vi "Begin.vi"(8 "error in":errorcluster) -> (0 "error out":errorcluster)   [LabVIEW 2016]
doc: "Called before other user functions, this VI is expected to open initial I/O refnums, load in file data, and do all program initialization. Notice that the <B>error out</B> terminal is simply used for data flow. Wiring it to other structures or subVIs ensures that this VI runs first."
uses:
  <vilib>/Rock Robotics/SystemInterfaces/spilib/spi_bus.ctl
  <vilib>/Rock Robotics/WPI/SPI/WPI_SPIMode.ctl
  <vilib>/Rock Robotics/SystemInterfaces/DIO/FPGA_DIOPWMChannel.ctl
  <vilib>/Rock Robotics/WPI/SafetyOutput/WPI_SafetyOutputConfigMenu.ctl
  <vilib>/Rock Robotics/WPI/DriverStation/WPI_DriverStationRobotMode2.ctl
  <vilib>/Rock Robotics/WPI/Joystick/WPI_JoystickDeviceEnum.ctl
  <vilib>/Rock Robotics/SystemInterfaces/DIO/FPGA_DIOChannel.ctl
  <vilib>/Rock Robotics/WPI/Encoder/WPI_EncoderType.ctl
  NI WPI/WPI_SerialPort_USB.ctl
  <vilib>/Rock Robotics/WPI/ThirdParty/CanMotor/TalonSRX/WPI_CANTalonSRX_APIControlMode.ctl
  <vilib>/Rock Robotics/WPI/Solenoid/WPI_SolenoidChannel.ctl
  <vilib>/Rock Robotics/SystemInterfaces/i2clib/i2c_bus.ctl
  <vilib>/Rock Robotics/WPI/Solenoid/WPI_SolenoidValue.ctl
  Robot Global Data.vi
  <vilib>/Rock Robotics/Network Tables/NT Write String Array.vi
  <vilib>/Rock Robotics/WPI/Counter/WPI_CounterDigitalInputToDigitalSource.vi
  navX Library v2/IO/Open/Z900_navX_Open_Serial.vi
  <vilib>/Rock Robotics/WPI/Solenoid/WPI_SolenoidOpenSingle.vi
  <vilib>/Rock Robotics/WPI/MotorControl/WPI_MotorControlOpen VictorSP.vi
  <vilib>/Rock Robotics/WPI/RobotDrive/WPI_RobotDriveOpen4MotorWithVictorSP.vi
  <vilib>/Rock Robotics/WPI/Solenoid/WPI_SolenoidSetEnum.vi
  navX Library v2/navX Library v2.lvlib
  NI WPI/NI WPI Serial USB.lvlib
panel:
  in  "Chip Select Active High (F)":bool
  in  "Mode (3)":T1=enum."Mode 3 (Clk Idle High,Sample on Trailing)"
  in  "Clock Rate (Hz)":dbl=500000.0
  in  "SPI Bus":T2=enum."SPI On-Board, CS1"
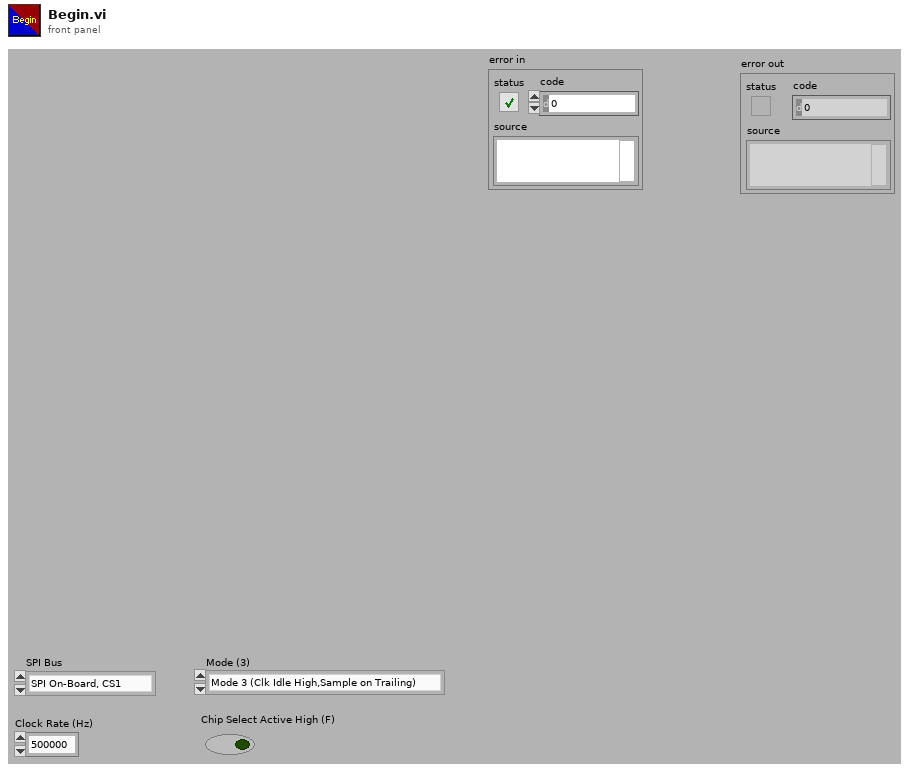
[diagram p1: front panel]
types:
  T1 = typedef "WPI_SPIMode.ctl" = enum16{"Mode 0 (Clk Idle Low,Sample on Leading)", "Mode 1 (Clk Idle Low,Sample on Trailing)", "Mode 2 (Clk Idle High,Sample on Leading)", "Mode 3 (Clk Idle High,Sample on Trailing)"}
  T2 = typedef "spi_bus.ctl" = enum16{"SPI On-Board, CS0", "SPI On-Board, CS1", "SPI On-Board, CS2", "SPI On-Board, CS3", "SPI MXP", "Invalid"}
  T3 = typedef "FPGA_DIOChannel.ctl" = enum8{"DIO 0", "DIO 1", "DIO 2", "DIO 3", "DIO 4", "DIO 5", "DIO 6", "DIO 7", "DIO 8", "DIO 9", "DIO MXP 0", "DIO MXP 1", "DIO MXP 2", "DIO MXP 3", "DIO MXP 4", "DIO MXP 5", "DIO MXP 6", "DIO MXP 7", "DIO MXP 8", "DIO MXP 9", "DIO MXP 10", "DIO MXP 11", "DIO MXP 12", "DIO MXP 13", "DIO MXP 14", "DIO MXP 15", "SPI Port CS1", "SPI Port CS2", "SPI Port CS3", "SPI Port MISO", "SPI Port MOSI", "Invalid"}
  T4 = typedef "WPI_SolenoidValue.ctl" = enum16{"Off", "On", "Forward", "Reverse"}
  T5 = typedef "i2c_bus.ctl" = enum16{"I2C On-Board", "I2C MXP", "Invalid"}
  T6 = typedef "WPI_SolenoidChannel.ctl" = enum8{"Solenoid 0", "Solenoid 1", "Solenoid 2", "Solenoid 3", "Solenoid 4", "Solenoid 5", "Solenoid 6", "Solenoid 7", "Invalid"}
  T7 = typedef "FPGA_DIOPWMChannel.ctl" = enum8{"PWM 0", "PWM 1", "PWM 2", "PWM 3", "PWM 4", "PWM 5", "PWM 6", "PWM 7", "PWM 8", "PWM 9", "PWM MXP 0", "PWM MXP 1", "PWM MXP 2", "PWM MXP 3", "PWM MXP 4", "PWM MXP 5", "PWM MXP 6", "PWM MXP 7", "PWM MXP 8", "PWM MXP 9", "Invalid"}
  T8 = typedef "WPI_JoystickDeviceEnum.ctl" = enum16{"USB 0", "USB 1", "USB 2", "USB 3", "USB 4", "USB 5"}
  T9 = typedef "WPI_CANTalonSRX_APIControlMode.ctl" = enum8{"Percent VBus", "Speed", "Position", "Slave", "Unchanged / Invalid", "Voltage Compensation", "Current", "Motion Profile", "Motion Magic"}
  T10 = typedef "NI WPI Serial USB.lvlib/WPI_SerialPort_USB.ctl" = enum16{"Onboard RS-232", "MXP TTL", "USB"}
  T11 = typedef "WPI_EncoderType.ctl" = enum16{"1x", "2x", "4x"}
  T12 = typedef "WPI_DriverStationRobotMode2.ctl" = enum16{"Autonomous Disabled", "Autonomous Enabled", "Teleop Disabled", "Teleop Enabled", "Disconnected", "Finish", "Test Disabled", "Test Enabled", "Emergency Stopped"}
  T13 = typedef "WPI_SafetyOutputConfigMenu.ctl" = enum16{"Enable", "Disable"}
  T14 = typedef "WPI_JoystickDevRef.ctl" = cluster{"Device":T8}
  T15 = typedef "WPI_I2CDevRef.ctl" = cluster{"DevStatus":errorcluster, "Device Address":u8, "Handle":i32, "I2C Bus":T5}
  T16 = typedef "WPI_MotorControlDeviceRef.ctl" = cluster{"DeviceStatus":errorcluster, "Type":T17, "PWM":cluster{"PWM Channel":T7, "DeadBand":T18}, "CAN":cluster{"Device Number":u8, "SetOutput VI Ref":variant, "GetOutput VI Ref":variant, "Enable VI Ref":variant, "Disable VI Ref":variant, "Data":variant}, "Invert":bool}
  T17 = typedef "WPI_MotorControlType.ctl" = enum16{"PWM", "CAN"}
  T18 = typedef "WPI_PWMDeadband.ctl" = cluster{"Name":string, "maxPositivePwm":i32, "minPositivePwm":i32, "centerPwm":i32, "maxNegativePwm":i32, "minNegativePwm":i32, "angularRange":u16}
  T19 = typedef "WPI_RobotDriveDevRef.ctl" = cluster{"DevStatus":errorcluster, "Motors[]":T16[], "Square Inputs":bool, "Max Output":dbl}
  T20 = typedef "WPI_SPIDevRef.ctl" = cluster{"DevStatus":errorcluster, "Handle":i32, "SPI Bus":T2}
  T21 = typedef "WPI_DigitalInputDevRef.ctl" = cluster{"DevStatus":errorcluster, "DIO Channel":T3}
  T22 = typedef "FPGA_CounterEncoderSourceConvertionLVSourceType.ctl" = cluster{"DevStatus":errorcluster, "AnalogTriggerMode?":bool, "DigitalMode":cluster{"DIO Channel":T23}, "AnalogTriggerMode":cluster{"AnalogTriggerIndex":T24, "OutputType":T25}}
  T23 = typedef "FPGA_DIODigitalSourceChannel.ctl" = enum8{"DIO 0", "DIO 1", "DIO 2", "DIO 3", "DIO 4", "DIO 5", "DIO 6", "DIO 7", "DIO 8", "DIO 9", "DIO MXP 0", "DIO MXP 1", "DIO MXP 2", "DIO MXP 3", "DIO MXP 4", "DIO MXP 5", "DIO MXP 6", "DIO MXP 7", "DIO MXP 8", "DIO MXP 9", "DIO MXP 10", "DIO MXP 11", "DIO MXP 12", "DIO MXP 13", "DIO MXP 14", "DIO MXP 15", "Disabled"}
  T24 = typedef "FPGA_AnalogTriggerIndex.ctl" = enum8{"Trig 0", "Trig 1", "Trig 2", "Trig 3", "Trig 4", "Trig 5", "Trig 6", "Trig 7", "Invalid"}
  T25 = typedef "FPGA_AnalogTriggerOutType.ctl" = enum16{"InWindow", "TriggerState", "Rising", "Falling"}
  T26 = typedef "WPI_EncoderDevRef.ctl" = cluster{"DevStatus":errorcluster, "EncoderIndex":T27, "CounterIndex":T28, "DistancePerCount":dbl, "Decoding Type":T11}
  T27 = typedef "FPGA_EncoderIdx.ctl" = enum8{"Enc 0", "Enc 1", "Enc 2", "Enc 3", "Enc 4", "Enc 5", "Enc 6", "Enc 7", "Invalid"}
  T28 = typedef "FPGA_CounterCtrSystemIndex.ctl" = enum8{"Ctr 0", "Ctr 1", "Ctr 2", "Ctr 3", "Ctr 4", "Ctr 5", "Ctr 6", "Ctr 7", "Invalid"}
  T29 = typedef "navX Library v2.lvlib/Z900_navX_DeviceTypeDef.ctl" = cluster{"Interface":cluster{"Protocol":T30, "Update Rate (4Hz-100Hz)":u8, "navX Open TypeDef":variant}, "Notify Packet":refnum<notifier>, "Loop VI Refnum":refnum<vi>, "Ready to Close Occurrence Refnum":refnum<k4>}
  T30 = typedef "navX Library v2.lvlib/Z900_navX_ProtocolTypeDef.ctl" = enum16{"SERIAL", "I2C", "SPI"}
  T31 = typedef "WPI_SolenoidDevRef.ctl" = cluster{"DevStatus":errorcluster, "Pneumatics Control Module":u8, "Forward Solenoid Channel":T6, "Reverse Solenoid Channel":T6}
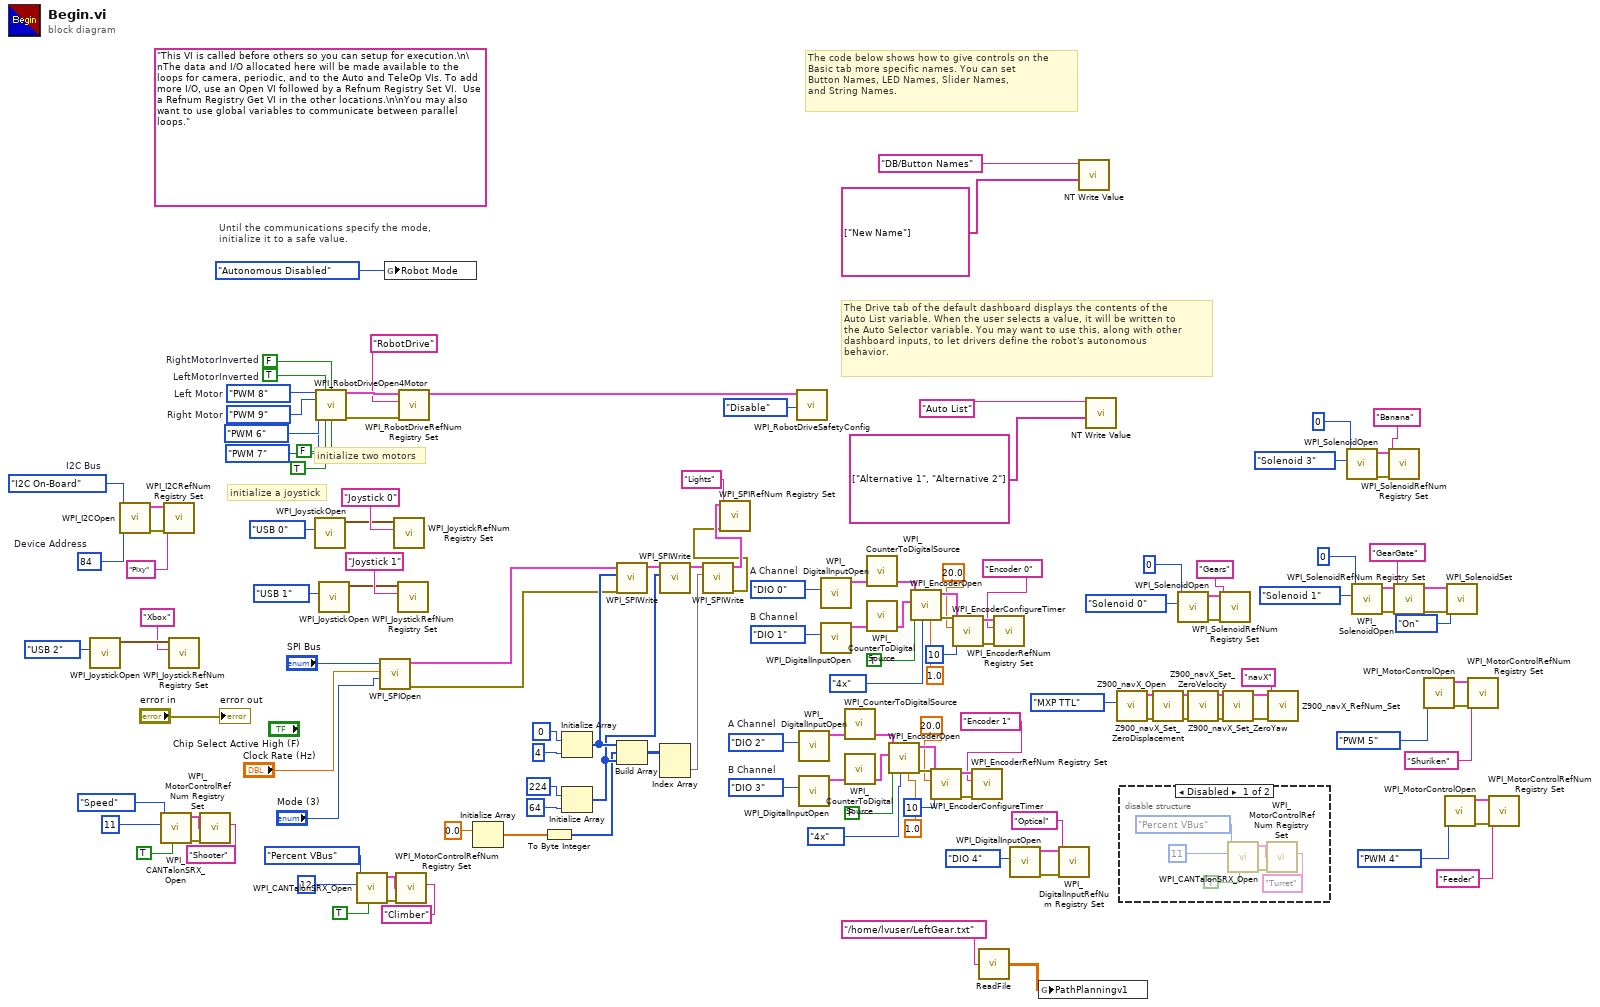
[diagram p0: block diagram]
diagram:
  w35 = u8 84  # Device Address
  w36 = i2c_bus."I2C On-Board"  # I2C Bus
  w103 = FPGA_DIOChannel."DIO 3"  # B Channel
  w102 = FPGA_DIOChannel."DIO 2"  # A Channel
  w119 = FPGA_DIOChannel."DIO 1"  # B Channel
  w118 = FPGA_DIOChannel."DIO 0"  # A Channel
  (unwired) "This VI is called before others so you can setup for execution.\n\nThe data and I/O allocated here will be made available to the loops for camera, periodic, and to the Auto and TeleOp VIs. To add more I/O, use an Open VI followed by a Refnum Registry Set VI.  Use a Refnum Registry Get VI in the other locations.\n\nYou may also want to use global variables to communicate between parallel loops."
  w134 = FPGA_DIOPWMChannel."PWM 9"  # Right Motor
  w135 = FPGA_DIOPWMChannel."PWM 8"  # Left Motor
  w139 = TRUE  # LeftMotorInverted
  w140 = FALSE  # RightMotorInverted
  # "The Drive tab of the default dashboard displays the contents of the\nAuto List variable. When the user selects a value, it will be written to\nthe Auto Selector variable. You may want to use this, along with other\ndashboard inputs, to let drivers define the robot's autonomous\nbehavior."
  # "The code below shows how to give controls on the\nBasic tab more specific names. You can set\nButton Names, LED Names, Slider Names,\nand String Names."
  # "initialize a joystick"
  # "Until the communications specify the mode,\ninitialize it to a safe value."
  # "initialize two motors"
  n1 = call <vilib>:"WPI_JoystickOpen.vi"("JoystickDevice"=WPI_JoystickDeviceEnum."USB 2") -> ("JoystickDevRef"=w49:T14)  [unwired: 10 in]
  n2 = call <vilib>:"WPI_I2COpen.vi"("Device Address"=w35, "I2C Bus"=w36) -> ("error out"=w34:errorcluster, "I2CDevRef"=w33:T15)  [unwired: 8 in]
  n3 = call <vilib>:"WPI_CANTalonSRX_Open.vi"("Invert"=TRUE, "Device Number"=11, "Control Mode"=WPI_CANTalonSRX_APIControlMode."Speed") -> ("error out"=w70:errorcluster, "CAN Talon SRX Ref"=w71:T16)  [unwired: 7 in]
  n4 = call <vilib>:"WPI_I2CRefNum Registry Set.vi"("error in (no error)"=w34, "refnum name"="Pixy", "I2CDevRef"=w33) -> ()  [unwired: 7 in, 2 out]
  n5 = call <vilib>:"WPI_JoystickRefNum Registry Set.vi"("refnum name"="Xbox", "JoystickDevRef"=w49) -> ()  [unwired: 8 in, 2 out]
  n6 = call <vilib>:"WPI_MotorControlRefNum Registry Set.vi"("error in (no error)"=w70, "refnum name"="Shooter", "MotorControlDevRef"=w71) -> ()  [unwired: 7 in, 2 out]
  n7 = call <vilib>:"WPI_JoystickOpen.vi"("JoystickDevice"=WPI_JoystickDeviceEnum."USB 0") -> ("JoystickDevRef"=w129:T14)  [unwired: 10 in]
  n8 = call-poly <vilib>:"WPI_RobotDriveOpen4Motor.vi"("Rear Left Motor"=w135, "Rear Left Motor Inverted"=w139, "Rear Right Motor Inverted"=w140, "Rear Right Motor"=w134, "Front Left Motor"=FPGA_DIOPWMChannel."PWM 6", "Front Right Motor"=FPGA_DIOPWMChannel."PWM 7", "Front Left Motor Inverted"=TRUE, "Front Right Motor Inverted"=FALSE) -> ("RobotDriveDevRef"=w138:T19, "error out"=w136:errorcluster)  [unwired: 6 in]
  n9 = call <vilib>:"WPI_JoystickOpen.vi"("JoystickDevice"=WPI_JoystickDeviceEnum."USB 1") -> ("JoystickDevRef"=w121:T14)  [unwired: 10 in]
  n10 = call <vilib>:"WPI_CANTalonSRX_Open.vi"("Invert"=TRUE, "Device Number"=12, "Control Mode"=WPI_CANTalonSRX_APIControlMode."Percent VBus") -> ("error out"=w64:errorcluster, "CAN Talon SRX Ref"=w65:T16)  [unwired: 7 in]
  n11 = call <vilib>:"WPI_SPIOpen.vi"("Mode (3)"="Mode (3)", "Clock Rate (Hz)"="Clock Rate (Hz)", "SPI Bus"="SPI Bus") -> ("error out"=w4:errorcluster, "SPIDevRef"=w5:T20)  [unwired: 7 in]
  n12 = global write "Robot Global Data.vi" "Robot Mode"(WPI_DriverStationRobotMode2."Autonomous Disabled" ("Robot Mode")) -> ()
  n13 = call <vilib>:"WPI_JoystickRefNum Registry Set.vi"("refnum name"="Joystick 0", "JoystickDevRef"=w129) -> ()  [unwired: 8 in, 2 out]
  n14 = call <vilib>:"WPI_MotorControlRefNum Registry Set.vi"("error in (no error)"=w64, "refnum name"="Climber", "MotorControlDevRef"=w65) -> ()  [unwired: 7 in, 2 out]
  n15 = call <vilib>:"WPI_JoystickRefNum Registry Set.vi"("refnum name"="Joystick 1", "JoystickDevRef"=w121) -> ()  [unwired: 8 in, 2 out]
  n16 = call <vilib>:"WPI_RobotDriveRefNum Registry Set.vi"("error in (no error)"=w136, "refnum name"="RobotDrive", "RobotDriveDevRef"=w138) -> ("RobotDriveDevRef"=w133:T19)  [unwired: 1 in, 7 out]
  n17 = Initialize Array(0.0 ("element")) -> (w9:dbl[])  [unwired: 1 in]
  n18 = To Byte Integer(number=w9) -> (8bit integer=w8:i8[])
  n19 = Initialize Array(u8 0 ("Data To Send"), u8 4 ("dimension size")) -> (w13:u8[])
  n20 = Initialize Array(u8 224 ("Data To Send"), u8 64 ("dimension size")) -> (w12:u8[])
  n21 = call <vilib>:"WPI_SPIWrite.vi"("error in (no error)"=w4, "Data To Send"=w13, "SPIDevRef"=w5) -> ("SPIDevRef"=w14:T20)  [unwired: 6 in, 2 out]
  n22 = Build Array(w13, w8, w12) -> (w7:u8[][])
  n23 = call <vilib>:"WPI_SPIWrite.vi"("Data To Send"=w12, "SPIDevRef"=w14) -> ("SPIDevRef"=w11:T20)  [unwired: 7 in, 2 out]
  n24 = Index Array(array=w7) -> (element=w6:u8[])  [unwired: 2 in]
  n25 = call <vilib>:"WPI_SPIWrite.vi"("Data To Send"=w6, "SPIDevRef"=w11) -> ("error out"=w1:errorcluster, "SPIDevRef"=w2:T20)  [unwired: 7 in, 1 out]
  n26 = call <vilib>:"WPI_SPIRefNum Registry Set.vi"("error in (no error)"=w1, "refnum name"="Lights", "SPIDevRef"=w2) -> ()  [unwired: 7 in, 2 out]
  n27 = call <vilib>:"WPI_RobotDriveSafetyConfig.vi"("mode"=WPI_SafetyOutputConfigMenu."Disable", "RobotDriveDevRef"=w133) -> ()  [unwired: 8 in, 2 out]
  n28 = call <vilib>:"WPI_DigitalInputOpen.vi"("DIO Channel"=w102) -> ("DigitalInputDevRef"=w99:T21)  [unwired: 1 in, 9 out]
  n29 = call <vilib>:"WPI_DigitalInputOpen.vi"("DIO Channel"=w103) -> ("DigitalInputDevRef"=w100:T21)  [unwired: 1 in, 9 out]
  n30 = call <vilib>:"WPI_DigitalInputOpen.vi"("DIO Channel"=w118) -> ("DigitalInputDevRef"=w115:T21)  [unwired: 1 in, 9 out]
  n31 = call <vilib>:"WPI_DigitalInputOpen.vi"("DIO Channel"=w119) -> ("DigitalInputDevRef"=w116:T21)  [unwired: 1 in, 9 out]
  n32 = call-poly <vilib>:"WPI_CounterToDigitalSource.vi"("DigitalInputDevRef"=w99) -> ("Digital Source"=w98:T22)  [unwired: 6 out]
  n33 = call-poly <vilib>:"WPI_CounterToDigitalSource.vi"("DigitalInputDevRef"=w100) -> ("Digital Source"=w101:T22)  [unwired: 6 out]
  n34 = call-poly <vilib>:"WPI_CounterToDigitalSource.vi"("DigitalInputDevRef"=w115) -> ("Digital Source"=w114:T22)  [unwired: 6 out]
  n35 = call-poly <vilib>:"WPI_CounterToDigitalSource.vi"("DigitalInputDevRef"=w116) -> ("Digital Source"=w117:T22)  [unwired: 6 out]
  n36 = call <vilib>:"WPI_EncoderOpen.vi"("DistancePerCount"=1.0, "Decoding Type"=WPI_EncoderType."4x", "Invert Direction (False)"=FALSE, "BSource"=w101, "ASource"=w98) -> ("error out"=w96:errorcluster, "EncoderDevRef"=w95:T26)  [unwired: 3 in, 2 out]
  n37 = call <vilib>:"WPI_EncoderOpen.vi"("DistancePerCount"=1.0, "Decoding Type"=WPI_EncoderType."4x", "Invert Direction (False)"=TRUE, "BSource"=w117, "ASource"=w114) -> ("error out"=w110:errorcluster, "EncoderDevRef"=w109:T26)  [unwired: 3 in, 2 out]
  n38 = call <vilib>:"WPI_EncoderConfigureTimer.vi"("error in (no error)"=w96, "Number Samples to Average"=u8 10, "Minimum Rate"=20.0, "EncoderDevRef"=w95) -> ("error out"=w92:errorcluster, "EncoderDevRef"=w91:T26)  [unwired: 6 in]
  n39 = call <vilib>:"WPI_EncoderConfigureTimer.vi"("error in (no error)"=w110, "Number Samples to Average"=u8 10, "Minimum Rate"=20.0, "EncoderDevRef"=w109) -> ("error out"=w106:errorcluster, "EncoderDevRef"=w105:T26)  [unwired: 6 in]
  n40 = call <vilib>:"WPI_EncoderRefNum Registry Set.vi"("error in (no error)"=w92, "refnum name"="Encoder 1", "EncoderDevRef"=w91) -> ()  [unwired: 7 in, 2 out]
  n41 = call "ReadFile.vi"("Name"="/home/lvuser/LeftGear.txt") -> ("Array - Numeric"=w29:dbl[][])
  n42 = call <vilib>:"WPI_EncoderRefNum Registry Set.vi"("error in (no error)"=w106, "refnum name"="Encoder 0", "EncoderDevRef"=w105) -> ()  [unwired: 7 in, 2 out]
  n43 = call <vilib>:"WPI_DigitalInputOpen.vi"("DIO Channel"=FPGA_DIOChannel."DIO 4") -> ("error out"=w25:errorcluster, "DigitalInputDevRef"=w24:T21)  [unwired: 9 in]
  n44 = global write "Robot Global Data.vi" "PathPlanningv1"(w29) -> ()
  n45 = call <vilib>:"WPI_DigitalInputRefNum Registry Set.vi"("error in (no error)"=w25, "refnum name"="Optical", "DigitalInputDevRef"=w24) -> ()  [unwired: 7 in, 2 out]
  n46 = call-poly <vilib>:"NT Write Value.vi"("String Array"=string[] ["New Name"], "Name"="DB/Button Names") -> ()  [unwired: 9 in, 1 out]
  n47 = call-poly <vilib>:"NT Write Value.vi"("String Array"=string[] ["Alternative 1", "Alternative 2"], "Name"="Auto List") -> ()  [unwired: 9 in, 1 out]
  n48 = call-poly "Z900_navX_Open.vi"("Serial Port"=WPI_SerialPort_USB."MXP TTL") -> ("error out"=w78:errorcluster, "navX Device"=w83:T29)  [unwired: 9 in]
  n49 = disable-structure shown="Disabled" {
    frame Disabled {
      n50 = call <vilib>:"WPI_CANTalonSRX_Open.vi"("Invert"=TRUE, "Device Number"=11, "Control Mode"=WPI_CANTalonSRX_APIControlMode."Percent VBus") -> ("error out"=w141:errorcluster, "CAN Talon SRX Ref"=w142:T16)  [unwired: 7 in]
      n51 = call <vilib>:"WPI_MotorControlRefNum Registry Set.vi"("error in (no error)"=w141, "refnum name"="Turret", "MotorControlDevRef"=w142) -> ()  [unwired: 7 in, 2 out]
    }
    frame Enabled {
    }
  }
  n52 = call "Z900_navX_Set_ZeroDisplacement.vi"("error in (no error)"=w78, "navX Device"=w83) -> ("error out"=w77:errorcluster, "navX Device"=w82:T29)  [unwired: 8 in]
  n53 = call-poly <vilib>:"WPI_SolenoidOpen.vi"("Solenoid Channel"=WPI_SolenoidChannel."Solenoid 0", "Pneumatics Control Module (0)"=u8 0) -> ("error out"=w63:errorcluster, "SolenoidDevRef"=w62:T31)  [unwired: 8 in]
  n54 = call "Z900_navX_Set_ZeroVelocity.vi"("error in (no error)"=w77, "navX Device"=w82) -> ("error out"=w76:errorcluster, "navX Device"=w81:T29)  [unwired: 8 in]
  n55 = call <vilib>:"WPI_SolenoidRefNum Registry Set.vi"("error in (no error)"=w63, "refnum name"="Gears", "SolenoidDevRef"=w62) -> ()  [unwired: 7 in, 2 out]
  n56 = call "Z900_navX_Set_ZeroYaw.vi"("error in (no error)"=w76, "navX Device"=w81) -> ("error out"=w79:errorcluster, "navX Device"=w80:T29)  [unwired: 8 in]
  n57 = call "Z900_navX_RefNum_Set.vi"("error in (no error)"=w79, "refnum name"="navX", "navX Device"=w80) -> ()  [unwired: 7 in, 2 out]
  n58 = call-poly <vilib>:"WPI_SolenoidOpen.vi"("Solenoid Channel"=WPI_SolenoidChannel."Solenoid 3", "Pneumatics Control Module (0)"=u8 0) -> ("error out"=w41:errorcluster, "SolenoidDevRef"=w40:T31)  [unwired: 8 in]
  n59 = call-poly <vilib>:"WPI_SolenoidOpen.vi"("Solenoid Channel"=WPI_SolenoidChannel."Solenoid 1", "Pneumatics Control Module (0)"=u8 0) -> ("error out"=w54:errorcluster, "SolenoidDevRef"=w53:T31)  [unwired: 8 in]
  n60 = call <vilib>:"WPI_SolenoidRefNum Registry Set.vi"("error in (no error)"=w41, "refnum name"="Banana", "SolenoidDevRef"=w40) -> ()  [unwired: 7 in, 2 out]
  n61 = call <vilib>:"WPI_SolenoidRefNum Registry Set.vi"("error in (no error)"=w54, "refnum name"="GearGate", "SolenoidDevRef"=w53) -> ("error out"=w28:errorcluster, "SolenoidDevRef"=w27:T31)  [unwired: 7 in]
  n62 = call-poly <vilib>:"WPI_MotorControlOpen.vi"("PWM Channel"=FPGA_DIOPWMChannel."PWM 5") -> ("error out"=w58:errorcluster, "MotorControlDeviceRef"=w57:T16)  [unwired: 9 in]
  n63 = call-poly <vilib>:"WPI_MotorControlOpen.vi"("PWM Channel"=FPGA_DIOPWMChannel."PWM 4") -> ("error out"=w46:errorcluster, "MotorControlDeviceRef"=w45:T16)  [unwired: 9 in]
  n64 = call-poly <vilib>:"WPI_SolenoidSet.vi"("error in (no error)"=w28, "Value"=WPI_SolenoidValue."On", "SolenoidDevRef"=w27) -> ()  [unwired: 7 in, 2 out]
  n65 = call <vilib>:"WPI_MotorControlRefNum Registry Set.vi"("error in (no error)"=w58, "refnum name"="Shuriken", "MotorControlDevRef"=w57) -> ()  [unwired: 7 in, 2 out]
  n66 = call <vilib>:"WPI_MotorControlRefNum Registry Set.vi"("error in (no error)"=w46, "refnum name"="Feeder", "MotorControlDevRef"=w45) -> ()  [unwired: 7 in, 2 out]
  "error out" <- "error in"
